vi "Configure Multi Turn Offset.vi"(0 "VISA resource name":refnum<visa-resource-name>, 5 "Motor ID (0)":u8, 7 "Multi Turn offset (0 deg)":dbl, 11 "error in (no error)":errorcluster) -> (4 "VISA resource name out":refnum<visa-resource-name>, 15 "error out":errorcluster)   [LabVIEW 2016, in "Dynamixel Motor.lvlib"]
doc: "Sets Multi Turn offset for the motor. This parameter is only valid for Multi Turn mode."
uses:
  Dynamixel Motor.lvlib
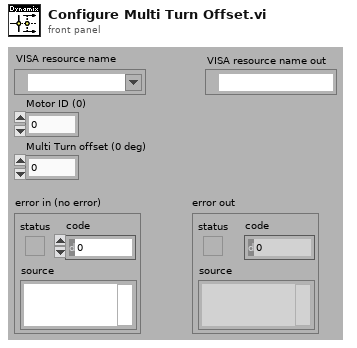
[diagram p1: front panel]
types:
  T1 = enum16{"big-endian, network order", "native, host order", "little-endian"}
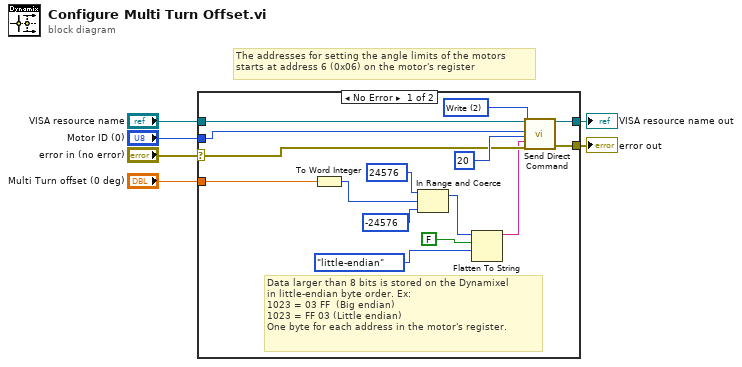
[diagram p0: block diagram]
diagram:
  # "The addresses for setting the angle limits of the motors\nstarts at address 6 (0x06) on the motor's register"
  n1 = case shown="No Error" "error in (no error)" {
    selector: "error in (no error)" -> [w15 w23]
    tunnel: [w18 w23] -> w5
    tunnel: "VISA resource name" -> [w21 w22]
    tunnel: [w19 w22] -> w3
    tunnel: "Motor ID (0)" -> [w17 _]
    tunnel: "Multi Turn offset (0 deg)" -> [w8 _]
    frame No Error {
      w20 = u16 2 items=["Ping", "Read", "Write", "Registered Write", "Action", "Reset", "Sync Write"] ("Select Action")
      # "Data larger than 8 bits is stored on the Dynamixel \nin little-endian byte order. Ex:\n1023 = 03 FF  (Big endian)\n1023 = FF 03 (Little endian)\nOne byte for each address in the motor's register."
      n2 = To Word Integer(number=w8) -> (16bit integer=w7:i16)
      n3 = In Range and Coerce(upper limit=i16 24576, x=w7, lower limit=i16 -24576) -> (coerced(x)=w11:i16)  [unwired: 1 out]
      n4 = Flatten To String(anything=w11, prepend array or string size? (T)=FALSE, byte order (0:big-endian, network order)=T1."little-endian") -> (data string=w12:string)  [unwired: 1 in, 2 out]
      n5 = call "Send Direct Command.vi"("VISA resource name"=w21, "Select Action"=w20, "Motor ID (0)"=w17, "Address"=u8 20, "Parameters"=w12, "Error in (no error)"=w15) -> ("VISA resource name out"=w19:refnum<visa-resource-name>, "Error out"=w18:errorcluster)  [unwired: 11 in, 1 out]
    }
    frame Error {
    }
  }
  "VISA resource name out" <- w3
  "error out" <- w5
